vi "Center Window.vi"(8 "error in (no error)":errorcluster, 9 "Height":i16, 10 "Width":i16, 11 "VI in":refnum<vi>) -> (0 "error out":errorcluster, 3 "VI out":refnum<vi>)   [LabVIEW 2020]
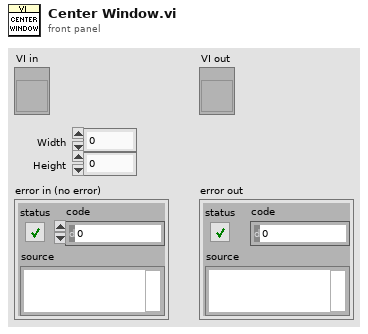
[diagram p1: front panel]
types:
  T1 = typedef "LVRectTypeDef.ctl" = cluster{"Left":i16, "Top":i16, "Right":i16, "Bottom":i16}
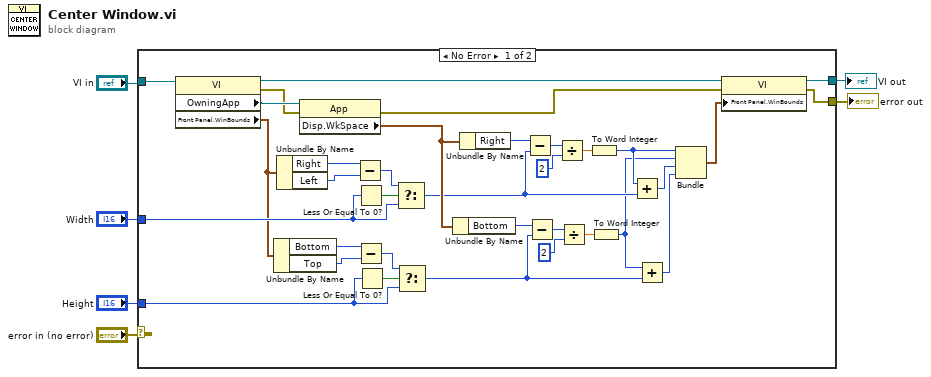
[diagram p0: block diagram]
diagram:
  n1 = case shown="No Error" "error in (no error)" {
    tunnel: "VI in" -> [w40 w41]
    tunnel: [w34 _] -> w5
    tunnel: [w36 w41] -> w6
    tunnel: "Width" -> [w29 _]
    tunnel: "Height" -> [w24 _]
    frame No Error {
      n2 = property class="VI"(reference=w40) -> (reference out=w37:refnum<vi>, error out=w38:errorcluster, "OwningApp"=w39:refnum<vi>, "Front Panel.WinBounds"=w8:T1)  [unwired: 1 in]
      n3 = Unbundle By Name(w8) -> ("Bottom"=w28:i16, "Top"=w27:i16)
      n4 = Unbundle By Name(w8) -> ("Right"=w33:i16, "Left"=w32:i16)
      n5 = property class="App"(reference=w39, error in=w38) -> (error out=w35:errorcluster, "Disp.WkSpace"=w19:T1)  [unwired: 1 out]
      n6 = Subtract(x=w33, y=w32) -> (x-y=w30:i16)
      n7 = Less Or Equal To 0?(x=w29) -> (x <= 0?=w31:bool)
      n8 = Subtract(x=w28, y=w27) -> (x-y=w25:i16)
      n9 = Less Or Equal To 0?(x=w24) -> (x <= 0?=w26:bool)
      n10 = Select(t=w30, s=w31, f=w29) -> (s? t:f=w13:i16)
      n11 = Select(t=w25, s=w26, f=w24) -> (s? t:f=w11:i16)
      n12 = Unbundle By Name(w19) -> ("Bottom"=w15:i16)
      n13 = Unbundle By Name(w19) -> ("Right"=w23:i16)
      n14 = Subtract(x=w23, y=w13) -> (x-y=w22:i16)
      n15 = Subtract(x=w15, y=w11) -> (x-y=w18:i16)
      n16 = Divide(x=w22, y=2) -> (x/y=w20:dbl)
      n17 = Divide(x=w18, y=2) -> (x/y=w16:dbl)
      n18 = To Word Integer(number=w20) -> (16bit integer=w14:i16)
      n19 = To Word Integer(number=w16) -> (16bit integer=w10:i16)
      n20 = Add(x=w14, y=w13) -> (x+y=w12:i16)
      n21 = Add(x=w10, y=w11) -> (x+y=w9:i16)
      n22 = Bundle(w14, w10, w12, w9) -> (w7:cluster{i16, i16, i16, i16})  [unwired: 1 in]
      n23 = property class="VI"(reference=w37, error in=w35, "Front Panel.WinBounds"=w7) -> (reference out=w36:refnum<vi>, error out=w34:errorcluster)
    }
    frame Error {
    }
  }
  "VI out" <- w6
  "error out" <- w5
